vi "GV RS sync.vi"() -> ()   [LabVIEW 2017]
panel:
  out "RS sync":bool
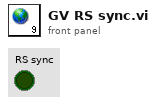
[diagram p1: front panel]
diagram:
